vi "Read TOML File (LV).vi"(7 "Default Value":variant, 8 "error in (no error)":errorcluster, 10 "BlueSerializer in":refnum<class "BlueSerializer.lvclass">, 11 "file path (use dialog)":path) -> (0 "error out":errorcluster, 3 "Value":variant)   [LabVIEW 2019, in "BlueTOMLSerializer.lvlib"]
uses:
  BlueTOMLSerializer.lvlib
  <userlib>/Blue Origin/BlueSerialization/BlueSerializer/BlueSerializer.lvclass
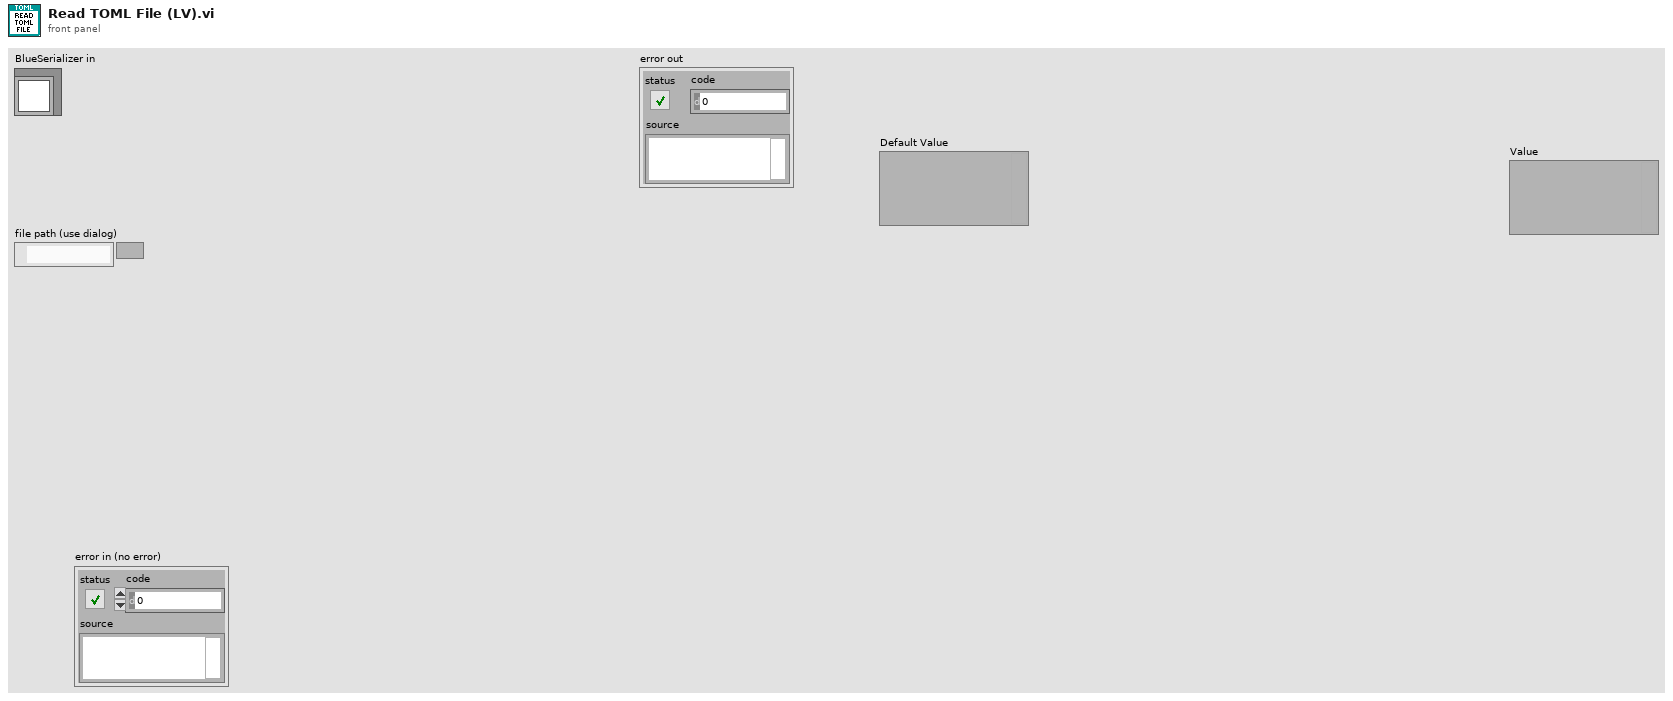
[diagram p1: front panel]
types:
  T1 = enum16{"open", "replace", "create", "open or create", "replace or create", "replace or create with confirmation"}
  T2 = typedef "BlueTOMLSerializer.lvlib/TOML Value.ctl" = cluster{"\\type":enum16{"Table", "Array", "String", "Integer", "Float", "Boolean", "Offset Date-Time", "Local Date-Time", "Local Date", "Local Time"}, "ÿýÿýÿýÿýÿýÿþÿýÿýÿý%LV-TOML.lvlib:TOML Key-Value Pair.ctlÿýÿýÿýÿýÿýÿþÿýÿýÿýLV-TOML.lvlib:TOML Value.ctl$":variant}
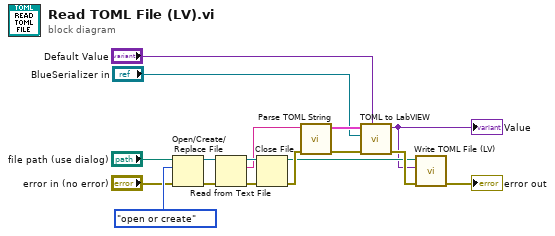
[diagram p0: block diagram]
diagram:
  n1 = Open/Create/Replace File(file path (use dialog)="file path (use dialog)", error in="error in (no error)", operation (0:open)=T1."open or create") -> (refnum out=w14:refnum<file>, error out=w15:errorcluster)  [unwired: 3 in, 1 out]
  n2 = Read from Text File(file (use dialog)=w14, error in=w15) -> (refnum out=w12:refnum<file>, text=w10:string, error out=w13:errorcluster)  [unwired: 2 in, 1 out]
  n3 = Close File(refnum=w12, error in=w13) -> (path=w4:path, error out=w9:errorcluster)
  n4 = call "Parse TOML String.vi"("error in (no error)"=w9, "String"=w10) -> ("error out"=w7:errorcluster, "Value"=w2:T2)  [unwired: 8 in]
  n5 = call "TOML to LabVIEW.vi"("Default Value"="Default Value", "error in (no error)"=w7, "BlueSerializer in"="BlueSerializer in", "TOML Value"=w2) -> ("error out"=w6:errorcluster, "LV Value"=w3:variant)  [unwired: 6 in]
  "Value" <- w3
  n6 = call "Write TOML File (LV).vi"("error in (no error)"=w6, "Value"=w3, "file path (use dialog)"=w4) -> ("error out"=→"error out":errorcluster)  [unwired: 8 in]
